vi "check_is_moving.vi"(8 "error in (no error)":errorcluster, 11 "ESP301viaTCPIP in":refnum<class "ESP301viaTCPIP.lvclass">) -> (0 "error out":errorcluster, 2 "Numeric":dbl, 3 "ESP301viaTCPIP out":refnum<class "ESP301viaTCPIP.lvclass">)   [LabVIEW 2019, in "ESP301viaTCPIP.lvlib" / "ESP301viaTCPIP.lvclass"]
uses:
  ESP301viaTCPIP.lvclass
  _stage/_stage.lvlibp/_stageClass/_stage.lvclass
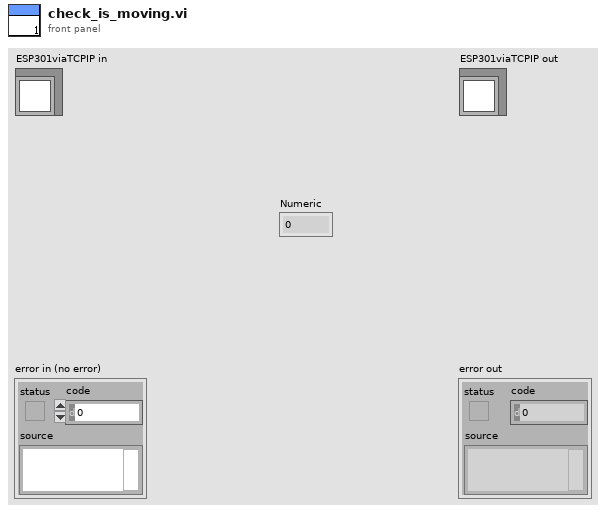
[diagram p1: front panel]
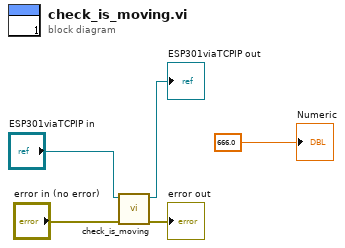
[diagram p0: block diagram]
diagram:
  n1 = call-parent "check_is_moving.vi"("error in (no error)"="error in (no error)", "_stage in"="ESP301viaTCPIP in") -> ("error out"=→"error out":errorcluster, "_stage out"=→"ESP301viaTCPIP out":refnum<class "ESP301viaTCPIP.lvclass">)  [unwired: 7 in, 1 out]
  "Numeric" <- 666.0
